vi "TCP Loop Async.vi"(7 "Secure":bool, 9 "Server URI":refnum<class "URI.lvclass">, 10 "TCP":refnum<k5>, 11 "Server in":refnum<class "Server.lvclass">) -> ()   [LabVIEW 2020, in "HTTP Server.lvlib" / "Server.lvclass"]
uses:
  Server.lvclass
  lv-uri/URI/URI/URI.lvclass
  lv-uri/URI/URI/URI.lvclass/URI.ctl
  lv-uri/URI/Build URI String.vi
  lv-uri/URI/Build Query String.vi
panel:
  out "URI String":string
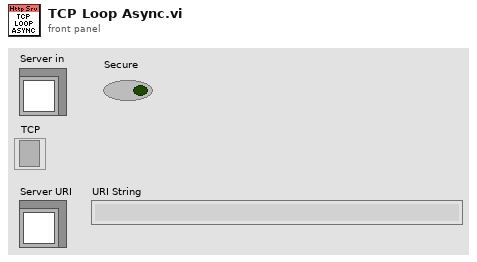
[diagram p1: front panel]
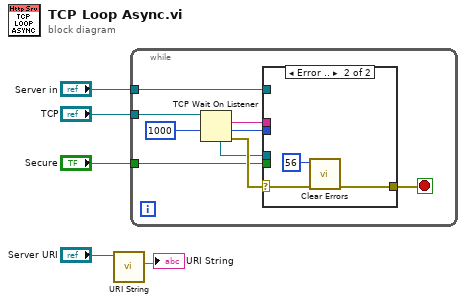
[diagram p0: block diagram]
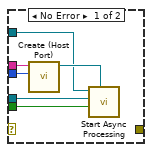
[diagram p2: hidden frame]
diagram:
  n1 = call "URI String.vi"("URI in"="Server URI") -> ("URI String"=→"URI String":string)  [unwired: 9 in, 1 out]
  n2 = while {
    tunnel: "TCP" -> [w14]
    tunnel: "Secure" -> [w8]
    tunnel: "Server in" -> [w7]
    stop <- w6 stop-if-true
    n3 = TCP Wait On Listener(9:1000 ("timeout ms (wait forever: -1)"), 11:w14) -> (0:w12:errorcluster, 1:w10:u16, 2:w9:string, 4:w11:refnum<k5>)  [unwired: 2 in, 1 out]
    n4 = case shown="Error .." w12 {
      selector: w12 -> [_ w23]
      tunnel: w11 -> [w20 _]
      tunnel: w10 -> [w18 _]
      tunnel: w9 -> [w17 _]
      tunnel: w8 -> [w19 _]
      tunnel: w7 -> [w15 _]
      tunnel: [_ w21] -> w6
      frame No Error {
        n5 = call "Create (Host Port).vi"("Port"=w18, "Host"=w17) -> ("URI out"=w16:refnum<class "URI.lvclass">)  [unwired: 9 in]
        n6 = call "Start Async Processing.vi"("Client URI"=w16, "Secure"=w19, "TCP"=w20, "Server in"=w15) -> ()  [unwired: 6 in, 2 out]
      }
      frame Error {
        n7 = call <vilib>:"Clear Errors.vi"("error in (no error)"=w23, "specific error code to clear (0: all)"=56) -> ("error out"=w21:errorcluster)  [unwired: 4 in, 1 out]
      }
    }
  }
